vi "ConfigureRange.vi"(0 "object in":refnum<class "AD2_MSO_SDK.lvclass">, 5 "error in (no error)":errorcluster) -> (14 "object out":refnum<class "AD2_MSO_SDK.lvclass">, 19 "error out":errorcluster)   [LabVIEW 2019, in "AD2_MSO_SDK.lvclass"]
uses:
  AD2_MSO_SDK.lvclass
  AD2_MSO_SDK.lvclass/AD2_MSO_SDK.ctl
  Olasdwf/Olasdwf.lvlib
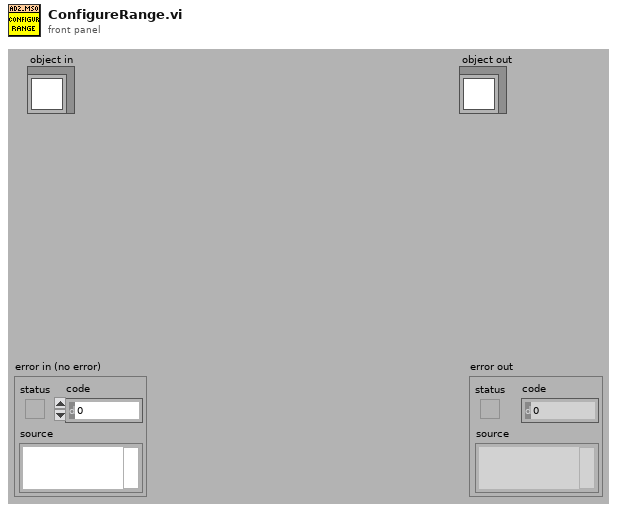
[diagram p1: front panel]
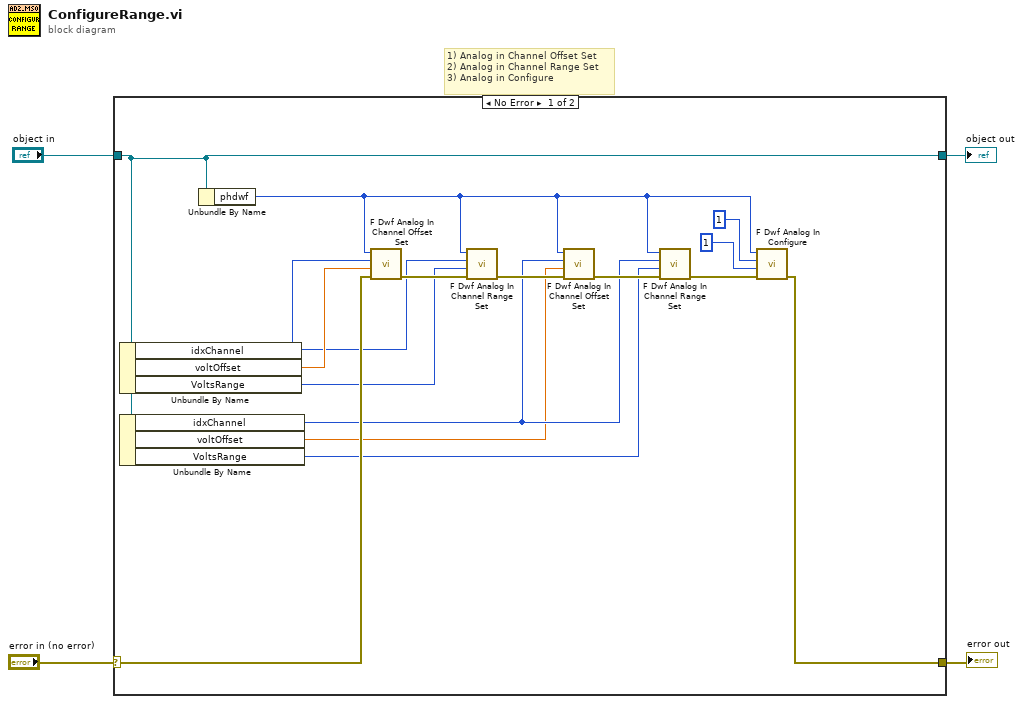
[diagram p0: block diagram]
diagram:
  # "1) Analog in Channel Offset Set\n2) Analog in Channel Range Set\n3) Analog in Configure"
  n1 = case shown="No Error" "error in (no error)" {
    selector: "error in (no error)" -> [w16 w22]
    tunnel: [w15 w22] -> w3
    tunnel: [w10 w21] -> w1
    tunnel: "object in" -> [w10 w21]
    frame No Error {
      n2 = Unbundle By Name(w10) -> ("idxChannel"=w12:i32, "voltOffset"=w13:dbl, "VoltsRange"=w11:u16)
      n3 = Unbundle By Name(w10) -> ("idxChannel"=w9:i32, "voltOffset"=w8:dbl, "VoltsRange"=w7:u16)
      n4 = Unbundle By Name(w10) -> ("phdwf"=w14:i32)
      n5 = call "F Dwf Analog In Channel Offset Set.vi"("error in (no error)"=w16, "voltOffset"=w13, "idxChannel"=w12, "hdwf"=w14) -> ("error out"=w20:errorcluster)  [unwired: 6 in, 1 out]
      n6 = call "F Dwf Analog In Channel Range Set.vi"("error in (no error)"=w20, "voltsRange"=w11, "idxChannel"=w12, "hdwf"=w14) -> ("error out"=w19:errorcluster)  [unwired: 6 in, 1 out]
      n7 = call "F Dwf Analog In Channel Offset Set.vi"("error in (no error)"=w19, "voltOffset"=w8, "idxChannel"=w9, "hdwf"=w14) -> ("error out"=w18:errorcluster)  [unwired: 6 in, 1 out]
      n8 = call "F Dwf Analog In Channel Range Set.vi"("error in (no error)"=w18, "voltsRange"=w7, "idxChannel"=w9, "hdwf"=w14) -> ("error out"=w17:errorcluster)  [unwired: 6 in, 1 out]
      n9 = call "F Dwf Analog In Configure.vi"("error in (no error)"=w17, "fStart"=1, "fReconfigure"=1, "hdwf"=w14) -> ("error out"=w15:errorcluster)  [unwired: 6 in, 1 out]
    }
    frame Error {
    }
  }
  "error out" <- w3
  "object out" <- w1
